vi "Fpga-MicroBlaze-Top.vi"() -> ()   [LabVIEW 2017]
uses:
  <vilib>/Platform/TimedLoop/XDataNode/timing_clust.ctl
  <vilib>/Platform/TimedLoop/XDataNode/nitl_modes.ctl
  <vilib>/Platform/TimedLoop/XDataNode/wakeup.ctl
  <vilib>/rvi/Emulation/niFpgaSctlEmulationGetInTimedLoop.vi
  <vilib>/rvi/Emulation/niFpgaEmulationReportErrorSimple.vi
  <vilib>/rvi/Emulation/niFpgaGetClockAttributes.vi
  <vilib>/rvi/Emulation/niFpgaCriticalErrorInLSC.vi
  <vilib>/rvi/eio/common/nirviEmuTemplateMethod_errors.vi
  <vilib>/rvi/interface/RandomDataEmulation/niFpgaRandomDataHandleErrors.vi
  <vilib>/Platform/TimedLoop/XDataNode/XDataNode.xnode
  <vilib>/eio/EIONode/EIONode.xnode
  <vilib>/rvi/DataTransferAndStorage/Container/XNode/niFpgaContainer.xnode
  <vilib>/rvi/interface/RandomDataEmulation/nirviRandomDataFpgaReadWriteTemplate.vi
  <vilib>/Platform/TimedLoop/XDataNode/XDNodeRunTimeDep.lvlib
panel:
  out "HeartBeat X 2":i16
  in  "HeartBeat":i16
  out "AXI_STR_RXD_tready 1":bool
  out "tvalid 1":bool
  out "tdata 1":u32
  out "tlast 1":bool
  out "AXI_STR_RXD_tready_Count 1":u16
  out "tvalid_Count 1":u16
  out "tlast_Count 1":u16
  out "tdata_LastNonZero 1":u32
  out "AXI_STR_RXD_tready 2":bool
  out "tvalid 2":bool
  out "tdata 2":u32
  out "tlast 2":bool
  out "AXI_STR_RXD_tready_Count 2":u16
  out "tvalid_Count 2":u16
  out "tlast_Count 2":u16
  out "tdata_LastNonZero 2":u32
  in  "Interrupt #1":bool
  in  "Interrupt #0":bool
  out "GPIO #2 out":u32
  in  "GPIO #2 in":u32
  out "GPIO #1 out":u32
  in  "GPIO #1 in":u32
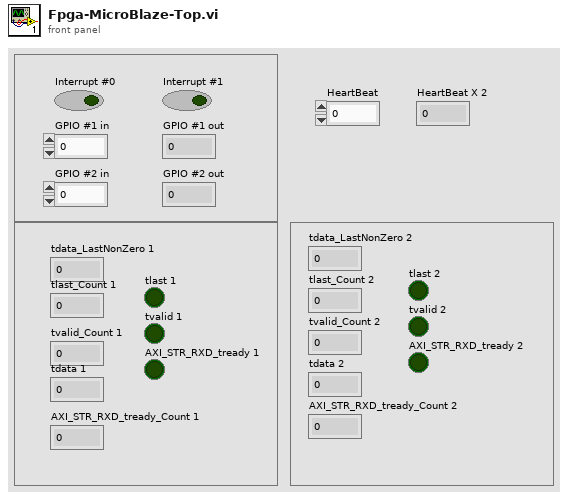
[diagram p1: front panel]
types:
  T1 = typedef "XDNodeRunTimeDep.lvlib/timing_clust.ctl" = cluster{"Expected End [f-1]":u64, "Actual End [f-1]":u64, "Finished Late? [f-1]":bool, "Expected End [i-1]":u64, "Actual End [i-1]":u64, "Finished Late? [i-1]":bool, "Expected Start [i]":u64, "Actual Start [i]":u64, "Expected Start [f]":u64, "Actual Start [f]":u64, "Source Name":string, "Structure Name":string, "Period":i64, "Deadline":i64, "Offset":i64, "Start":i64, "Priority":i32, "Timeout":i32, "Mode":T2, "Wakeup Reason":T3, "Error":errorcluster, "Source Type":string, "Secondary Source Type":string, "Global End Time":u64, "Global Start Time":u64, "Frame Duration":u64, "Iteration Duration":u64, "Assigned CPU":i32, "I/O Scan Engine Mode":u32}
  T2 = typedef "XDNodeRunTimeDep.lvlib/nitl_modes.ctl" = enum32{"No Change", "Process missed periods, maintain original phase", "Discard missed periods, maintain original phase", "Process missed periods, ignore original phase", "Discard missed periods, ignore original phase"}
  T3 = typedef "XDNodeRunTimeDep.lvlib/wakeup.ctl" = enum32{"Normal", "Aborted", "Asynchronous wakeup", "Timing source error", "Timed loop error", "Timeout"}
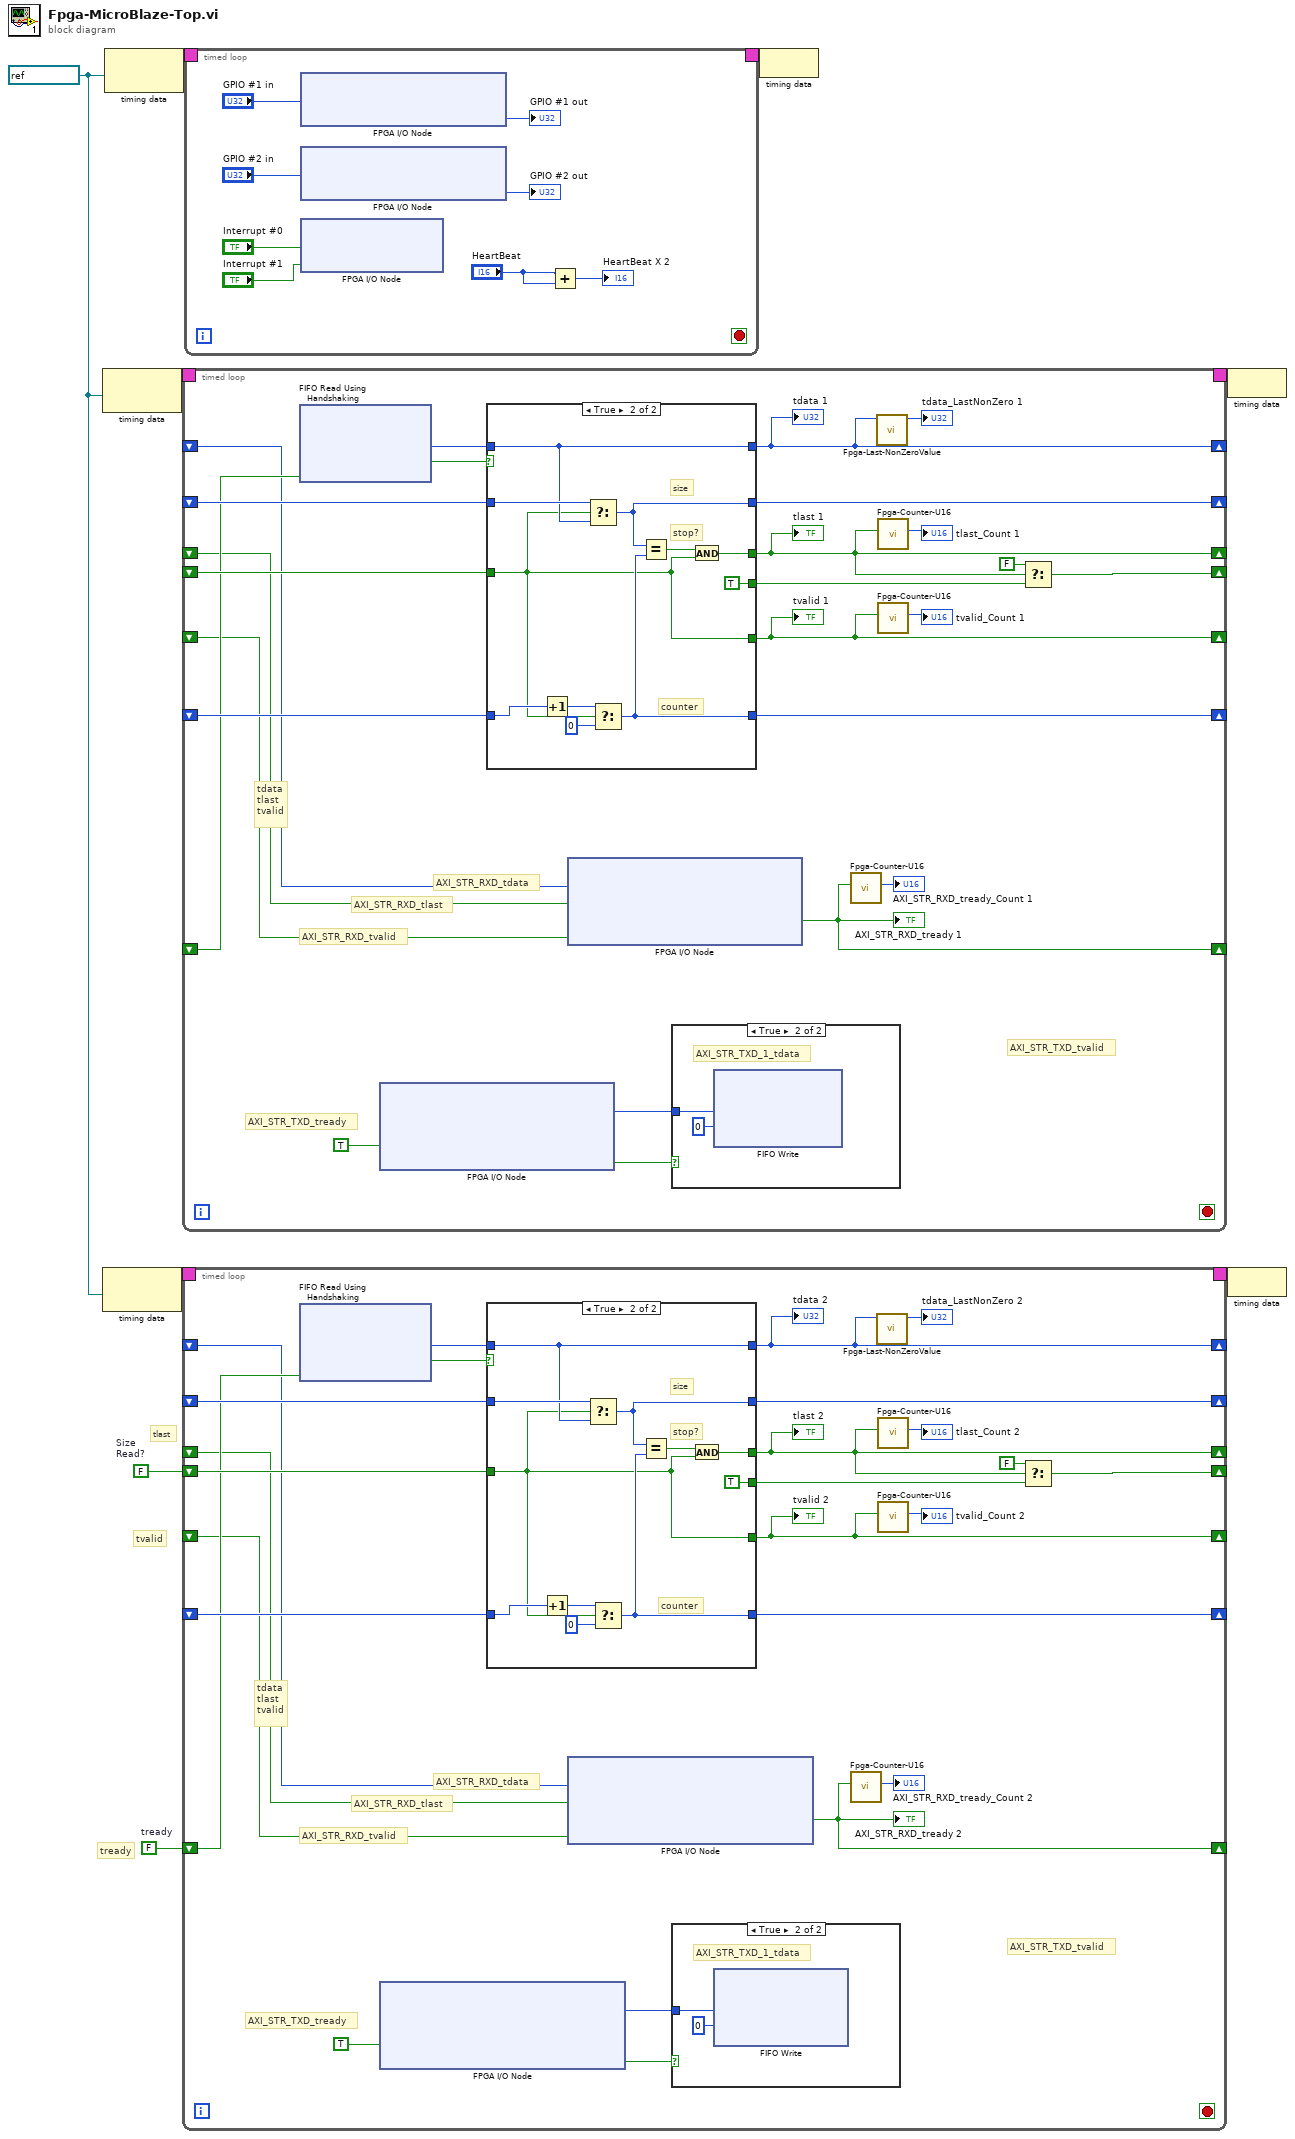
[diagram p0: block diagram]
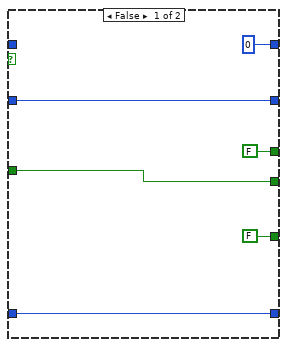
[diagram p3: hidden frame]
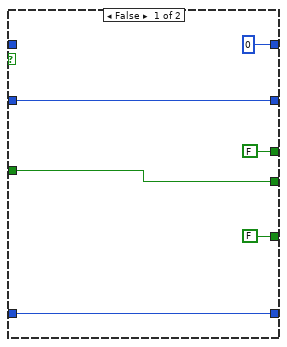
[diagram p5: hidden frame]
diagram:
  w4 = FALSE  # Size Read?
  w5 = FALSE  # tready
  w1 = refnum<k21> "100MHz" ("Source Name")
  # "tlast"
  # "tvalid"
  # "tready"
  n1 = node-c288(w1) -> (w3:T1)
  n2 = node-c288(w1) -> (w7:T1)
  n3 = node-c288(w1) -> (w9:T1)
  n4 = timed-loop {
    timing: w3 -> [_]
    timing-out: [_] -> w2
    shift-right: [w15] -> _
    shift-left: _ -> [w33]
    shift-right: [w30] -> _
    shift-left: _ -> [w32]
    shift-right: [w28] -> _
    shift-left: _ -> [w29]
    shift-right: [w11] -> _
    shift-left: _ -> [w21]
    shift-right: [w10] -> _
    shift-left: _ -> [w27]
    shift-right: [w25] -> _
    shift-left: _ -> [w23]
    shift-right: [w14] -> _
    shift-left: _ -> [w22]
    stop <- _ stop-if-true
    # "AXI_STR_TXD_tvalid"
    # "AXI_STR_TXD_tready"
    # "AXI_STR_RXD_tvalid"
    # "AXI_STR_RXD_tlast"
    # "AXI_STR_RXD_tdata"
    # "tdata\ntlast\ntvalid"
    n5 = xnode ("FIFO Read Using Handshaking")("Ready for Output"=w27) -> ("Element"=w31:u32, "Output Valid"=w34:bool)  [unwired: 1 in, 1 out]
    n6 = xnode "FPGA I/O Node"("d_microblaze_i\\AXI_STR_TXD_tready"=TRUE ("d_microblaze\\AXI_STR_TXD_tready")) -> ("d_microblaze_i\\AXI_STR_TXD_tdata"=w18:u32, "d_microblaze_i\\AXI_STR_TXD_tvalid"=w19:bool)  [unwired: 4 in, 5 out]
    n7 = case shown="True" w34 {
      tunnel: w33 -> [w41 w43]
      tunnel: [w41 TRUE ("Size\nRead?")] -> w16
      tunnel: w32 -> [w42 w53]
      tunnel: w31 -> [_ w48]
      tunnel: [w42 w47] -> w30
      tunnel: w29 -> [w40 w52]
      tunnel: [w40 w46] -> w28
      tunnel: [FALSE ("Size\nRead?") w43] -> w11
      tunnel: [u32 0 ("Element") w48] -> w25
      tunnel: [FALSE w44] -> w14
      frame False {
      }
      frame True {
        # "stop?"
        # "size"
        # "counter"
        n8 = Increment(x=w52) -> (x+1=w50:u32)
        n9 = Select(t=w53, s=w43, f=w48) -> (s? t:f=w47:u32)
        n10 = Select(t=w50, s=w43, f=u32 0) -> (s? t:f=w46:u32)
        n11 = Equal?(x=w47, y=w46) -> (x = y?=w45:bool)
        n12 = And(x=w45, y=w43) -> (x .and. y?=w44:bool)
      }
    }
    "tvalid 1" <- w11
    "tdata 1" <- w25
    "tlast 1" <- w14
    n13 = xnode "FPGA I/O Node"("d_microblaze_i\\AXI_STR_RXD_tdata"=w23, "d_microblaze_i\\AXI_STR_RXD_tlast"=w22, "d_microblaze_i\\AXI_STR_RXD_tvalid"=w21) -> ("d_microblaze_i\\AXI_STR_RXD_tready"=w10:bool)  [unwired: 4 in, 4 out]
    "AXI_STR_RXD_tready 1" <- w10
    n14 = case shown="True" w19 {
      tunnel: w18 -> [_ w36]
      frame False {
      }
      frame True {
        # "AXI_STR_TXD_1_tdata"
        n15 = xnode ("FIFO Write")("Element"=w36, "Timeout"=0) -> ()  [unwired: 1 in, 2 out]
      }
    }
    n16 = call "Fpga-Counter-U16.vi"("d_mcs_i\\IO_BUS_read_strobe"=w10) -> ("Numeric"=→"AXI_STR_RXD_tready_Count 1":u16)  [unwired: 10 in]
    n17 = call "Fpga-Last-NonZeroValue.vi"("d_mcs_i\\IO_BUS_write_data in"=w25) -> ("d_mcs_i\\IO_BUS_write_data out"=→"tdata_LastNonZero 1":u32)  [unwired: 10 in]
    n18 = call "Fpga-Counter-U16.vi"("d_mcs_i\\IO_BUS_read_strobe"=w14) -> ("Numeric"=→"tlast_Count 1":u16)  [unwired: 10 in]
    n19 = call "Fpga-Counter-U16.vi"("d_mcs_i\\IO_BUS_read_strobe"=w11) -> ("Numeric"=→"tvalid_Count 1":u16)  [unwired: 10 in]
    n20 = Select(t=FALSE, s=w14, f=w16) -> (s? t:f=w15:bool)
  }
  n21 = timed-loop {
    timing: w7 -> [_]
    timing-out: [_] -> w6
    shift-right: [w61] -> _
    shift-left: w4 -> [w79]
    shift-right: [w76] -> _
    shift-left: _ -> [w78]
    shift-right: [w74] -> _
    shift-left: _ -> [w75]
    shift-right: [w57] -> _
    shift-left: _ -> [w67]
    shift-right: [w56] -> _
    shift-left: w5 -> [w73]
    shift-right: [w71] -> _
    shift-left: _ -> [w69]
    shift-right: [w60] -> _
    shift-left: _ -> [w68]
    stop <- _ stop-if-true
    # "AXI_STR_TXD_tvalid"
    # "AXI_STR_TXD_tready"
    # "AXI_STR_RXD_tvalid"
    # "AXI_STR_RXD_tlast"
    # "AXI_STR_RXD_tdata"
    # "tdata\ntlast\ntvalid"
    n22 = xnode ("FIFO Read Using Handshaking")("Ready for Output"=w73) -> ("Element"=w77:u32, "Output Valid"=w80:bool)  [unwired: 1 in, 1 out]
    n23 = xnode "FPGA I/O Node"("d_microblaze_i\\AXI_STR_TXD_1_tready"=TRUE ("d_microblaze\\AXI_STR_TXD_tready")) -> ("d_microblaze_i\\AXI_STR_TXD_1_tdata"=w64:u32, "d_microblaze_i\\AXI_STR_TXD_1_tvalid"=w65:bool)  [unwired: 4 in, 5 out]
    n24 = case shown="True" w80 {
      tunnel: w79 -> [w87 w89]
      tunnel: [w87 TRUE ("Size\nRead?")] -> w62
      tunnel: w78 -> [w88 w99]
      tunnel: w77 -> [_ w94]
      tunnel: [w88 w93] -> w76
      tunnel: w75 -> [w86 w98]
      tunnel: [w86 w92] -> w74
      tunnel: [FALSE ("Size\nRead?") w89] -> w57
      tunnel: [u32 0 ("Element") w94] -> w71
      tunnel: [FALSE w90] -> w60
      frame False {
      }
      frame True {
        # "stop?"
        # "size"
        # "counter"
        n25 = Increment(x=w98) -> (x+1=w96:u32)
        n26 = Select(t=w99, s=w89, f=w94) -> (s? t:f=w93:u32)
        n27 = Select(t=w96, s=w89, f=u32 0) -> (s? t:f=w92:u32)
        n28 = Equal?(x=w93, y=w92) -> (x = y?=w91:bool)
        n29 = And(x=w91, y=w89) -> (x .and. y?=w90:bool)
      }
    }
    "tvalid 2" <- w57
    "tdata 2" <- w71
    "tlast 2" <- w60
    n30 = xnode "FPGA I/O Node"("d_microblaze_i\\AXI_STR_RXD_1_tdata"=w69, "d_microblaze_i\\AXI_STR_RXD_1_tlast"=w68, "d_microblaze_i\\AXI_STR_RXD_1_tvalid"=w67) -> ("d_microblaze_i\\AXI_STR_RXD_1_tready"=w56:bool)  [unwired: 4 in, 4 out]
    "AXI_STR_RXD_tready 2" <- w56
    n31 = case shown="True" w65 {
      tunnel: w64 -> [_ w82]
      frame False {
      }
      frame True {
        # "AXI_STR_TXD_1_tdata"
        n32 = xnode ("FIFO Write")("Element"=w82, "Timeout"=0) -> ()  [unwired: 1 in, 2 out]
      }
    }
    n33 = call "Fpga-Counter-U16.vi"("d_mcs_i\\IO_BUS_read_strobe"=w56) -> ("Numeric"=→"AXI_STR_RXD_tready_Count 2":u16)  [unwired: 10 in]
    n34 = call "Fpga-Last-NonZeroValue.vi"("d_mcs_i\\IO_BUS_write_data in"=w71) -> ("d_mcs_i\\IO_BUS_write_data out"=→"tdata_LastNonZero 2":u32)  [unwired: 10 in]
    n35 = call "Fpga-Counter-U16.vi"("d_mcs_i\\IO_BUS_read_strobe"=w60) -> ("Numeric"=→"tlast_Count 2":u16)  [unwired: 10 in]
    n36 = call "Fpga-Counter-U16.vi"("d_mcs_i\\IO_BUS_read_strobe"=w57) -> ("Numeric"=→"tvalid_Count 2":u16)  [unwired: 10 in]
    n37 = Select(t=FALSE, s=w60, f=w62) -> (s? t:f=w61:bool)
  }
  n38 = timed-loop {
    timing: w9 -> [_]
    timing-out: [_] -> w8
    stop <- _ stop-if-true
    n39 = xnode "FPGA I/O Node"("d_microblaze_i\\gpio_rtl_tri_i"="GPIO #1 in") -> ("d_microblaze_i\\gpio_rtl_0_tri_o"=→"GPIO #1 out":u32)  [unwired: 2 in, 2 out]
    n40 = xnode "FPGA I/O Node"("d_microblaze_i\\gpio_rtl_1_tri_i"="GPIO #2 in") -> ("d_microblaze_i\\gpio_rtl_2_tri_o"=→"GPIO #2 out":u32)  [unwired: 2 in, 2 out]
    n41 = xnode "FPGA I/O Node"("d_microblaze_i\\In0"="Interrupt #0", "d_microblaze_i\\In1"="Interrupt #1") -> ()  [unwired: 2 in, 2 out]
    n42 = Add(x="HeartBeat", y="HeartBeat") -> (x+y=→"HeartBeat X 2":i16)
  }
  n43 = node-c288(w8) -> ()
  n44 = node-c288(w2) -> ()
  n45 = node-c288(w6) -> ()
